vi "EasyDAQx1.vi"() -> ()   [LabVIEW 2011]
panel:
  in  "Show cursor":bool
  out "?":dbl
  out "?":waveform(dbl)(graph)
  in  "Set DAC":bool
  in  "Output (Volts) 2":sgl(slide) caption="Output (Volts)" min=-4.096 max=4.096 step=0.001 scale=-4.096..4.096 scale format="%#.2f"
  out "Numeric":i32
  out "Offsets":dbl[](array[numeric])
  out "Gains":dbl[](array[numeric])
  out "Gain 5":i32
  out "P-Channel":i32
  out "NumBytes":i32
  out "N-channel":i32
  out "NumChannel":i32
  in  "Quit":bool
  out "connected to device":bool
  in  "VISA resource Input":refnum<visa-resource-name>
  in  "Rate (ms)":dbl=500.0 min=10.0 max=65535.0 step=10.0
  out "Final Value":dbl
  in  "Offset":dbl
  in  "Gain":dbl
  out "Voltage":dbl
  in  "OK Button":bool
  in  "?":bool
  in  "Range":string(combo)="1"
  in  "Ch-":string(combo)="0"
  in  "Ch+":string(combo)="7"
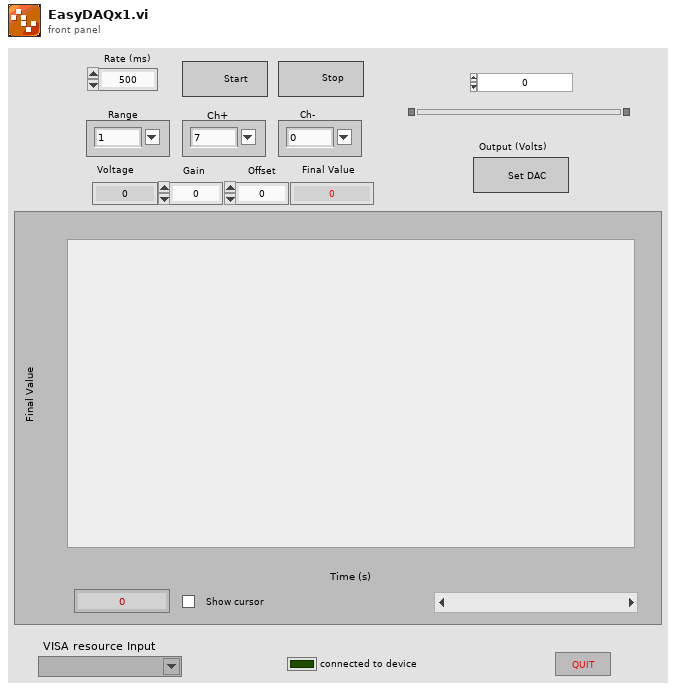
[diagram p1: front panel]
types:
  T1 = enum8{"Enabled", "Disabled", "Disabled and Grayed Out"}
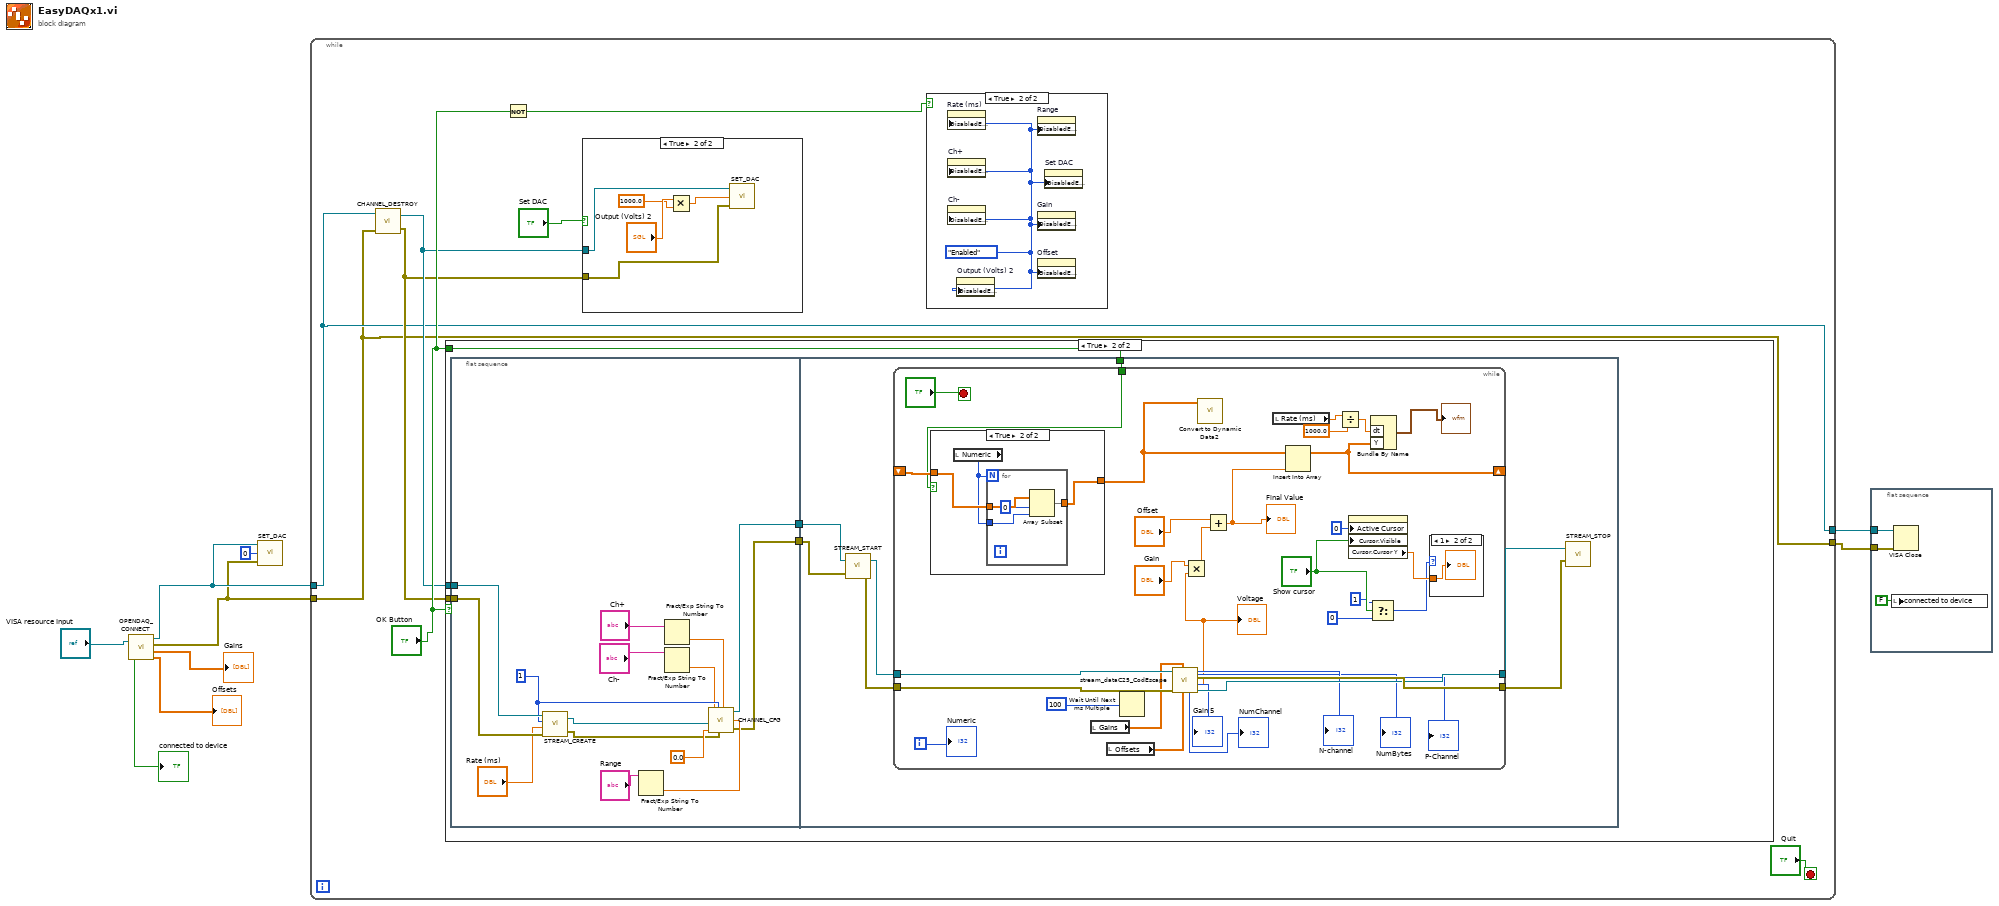
[diagram p0: block diagram]
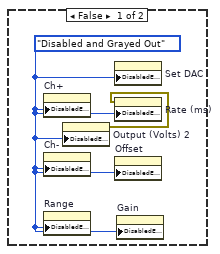
[diagram p3: hidden frame]
diagram:
  n1 = call "OPENDAQ_CONNECT.vi"("VISA resourceINPUT"="VISA resource Input") -> ("connected to device"=→"connected to device":bool, "VISA resource Salida"=w3:refnum<visa-resource-name>, "error out"=w2:errorcluster, "Gains"=→"Gains":dbl[], "Offsets"=→"Offsets":dbl[])
  n2 = call "SET_DAC.vi"("error in (no error)"=w2, "Input"=0, "VISA resource Input"=w3) -> ()  [unwired: 2 out]
  n3 = while {
    tunnel: w3 -> [w11]
    tunnel: w2 -> [w10]
    tunnel: [w11] -> w9
    tunnel: [w10] -> w8
    stop <- "Quit" stop-if-true
    n4 = call "CHANNEL_DESTROY.vi"("error INPUT"=w10, "VISA resource Input"=w11) -> ("error out"=w13:errorcluster, "VISA resource name out"=w14:refnum<visa-resource-name>)  [unwired: 1 in]
    n5 = case shown="True" "OK Button" {
      tunnel: w14 -> [_ w30]
      tunnel: w13 -> [_ w29]
      tunnel: "OK Button" -> [_ w26]
      frame False {
      }
      frame True {
        n6 = flat-sequence {
          tunnel: w30 -> [w45]
          tunnel: w29 -> [w44]
          tunnel: [w32] -> w28
          tunnel: [w31] -> w27
          tunnel: w28 -> [w48]
          tunnel: w27 -> [w47]
          tunnel: w26 -> [w46]
          frame #0 {
            w41 = i8 1 ("Channel")
            n7 = call "STREAM_CREATE.vi"("error in (no error)"=w44, "Period"="Rate (ms)", "Channel"=w41, "VISA resource Input"=w45) -> ("error out"=w39:errorcluster, "VISA resource name out"=w42:refnum<visa-resource-name>)
            n8 = Fract/Exp String To Number(string="Range") -> (number=w33:dbl)  [unwired: 3 in, 1 out]
            n9 = Fract/Exp String To Number(string="Ch+") -> (number=w37:dbl)  [unwired: 3 in, 1 out]
            n10 = Fract/Exp String To Number(string="Ch-") -> (number=w35:dbl)  [unwired: 3 in, 1 out]
            n11 = call "CHANNEL_CFG.vi"("Pchan"=w37, "Channel"=w41, "Nchan"=w35, "VISA resource name"=w42, "error in (no error)"=w39, "Mode"=0.0, "Gain"=w33) -> ("VISA resource name out"=w32:refnum<visa-resource-name>, "error out"=w31:errorcluster)
          }
          frame #1 {
            n12 = call "STREAM_START.vi"("error in (no error)"=w47, "VISA resource name"=w48) -> ("error out"=w52:errorcluster, "VISA resource name out"=w51:refnum<visa-resource-name>)
            n13 = while {
              tunnel: w51 -> [w84]
              tunnel: w52 -> [w83]
              tunnel: [w81] -> w50
              tunnel: [w82] -> w49
              shift-right: [w63] -> _
              shift-left: _ -> [w75]
              tunnel: w46 -> [w71]
              i -> [w69]
              stop <- "?" stop-if-true
              n14 = case shown="True" w71 {
                tunnel: w75 -> [w87 w90]
                tunnel: [w87 w89] -> w70
                frame False {
                }
                frame True {
                  n15 = local read "Numeric"() -> (w88:i32)
                  n16 = for {
                    N: w88 -> [_]
                    tunnel: w90 -> [w94]
                    tunnel: [w92] -> w89
                    tunnel: w88 -> [w91]
                    n17 = Array Subset(array=w94, index=0, length=w91) -> (w92:dbl[])
                  }
                }
              }
              n18 = local read "Gains"() -> (w74:dbl[])
              n19 = local read "Offsets"() -> (w73:dbl[])
              n20 = Wait Until Next ms Multiple(millisecond multiple=u32 100) -> ()  [unwired: 1 out]
              n21 = call "stream_dataC25_CodEscape.vi"("Offsets"=w73, "Gains"=w74, "error out 2"=w83, "VISA resource name out 2"=w84) -> ("VISA resource name out"=w81:refnum<visa-resource-name>, "DATA"=w67:dbl, "P-Channel"=→"P-Channel":i32, "N-channel"=→"N-channel":i32, "NumChannel"=→"NumChannel":i32, "NumBytes"=→"NumBytes":i32, "Gain"=→"Gain 5":i32, "error out"=w82:errorcluster)
              "Voltage" <- w67
              n22 = Multiply(x="Gain", y=w67) -> (x*y=w66:dbl)
              n23 = call "Convert to Dynamic Data2"("Array"=w70) -> ()  [unwired: 3 in, 1 out]
              n24 = Add(x="Offset", y=w66) -> (x+y=w64:dbl)
              "Final Value" <- w64
              n25 = local read "Rate (ms)"() -> (w61:dbl)
              n26 = Insert Into Array(array=w70, new element=w64) -> (w63:dbl[])  [unwired: 1 in]
              n27 = Divide(x=w61, y=1000.0) -> (x/y=w62:dbl)
              n28 = property class="WFGraph (strict)"("Active Cursor"=u32 0, "Cursor.Visible"="Show cursor") -> ("Cursor.Cursor Y"=w56:dbl)  [unwired: 2 in, 2 out]
              n29 = Bundle By Name("dt"=w62, "Y"=w63) -> (→"?":waveform(dbl))  [unwired: 1 in]
              n30 = Select(t=u8 1 ("Disabled"), s="Show cursor", f=u8 0 ("Disabled")) -> (s? t:f=w54:u8)
              n31 = case shown="1" w54 {
                tunnel: w56 -> [_ w86]
                frame 0, Default {
                }
                frame 1 {
                  "?" <- w86
                }
              }
              "Numeric" <- w69
            }
            n32 = call "STREAM_STOP.vi"("error in (no error)"=w49, "VISA resource name"=w50) -> ()  [unwired: 2 out]
          }
        }
      }
    }
    n33 = Not(x="OK Button") -> (.not. x?=w15:bool)
    n34 = case shown="True" "Set DAC" {
      tunnel: w14 -> [_ w22]
      tunnel: w13 -> [_ w21]
      frame False {
      }
      frame True {
        n35 = Multiply(x="Output (Volts) 2", y=sgl 1000.0) -> (x*y=w18:sgl)
        n36 = call "SET_DAC.vi"("error in (no error)"=w21, "Input"=w18, "VISA resource Input"=w22) -> ()  [unwired: 2 out]
      }
    }
    n37 = case shown="True" w15 {
      frame False {
        w23 = T1."Disabled and Grayed Out" ("Disabled")
        n38 = property on="Ch+" class="CmbBox"("DisabledEnum"=w23) -> ()  [unwired: 2 in, 2 out]
        n39 = property on="Ch-" class="CmbBox"("DisabledEnum"=w23) -> ()  [unwired: 2 in, 2 out]
        n40 = property on="Range" class="CmbBox"("DisabledEnum"=w23) -> ()  [unwired: 2 in, 2 out]
        n41 = property on="Output (Volts) 2" class="Slide (strict)"("DisabledEnum"=w23) -> (error out=w24:errorcluster)  [unwired: 2 in, 1 out]
        n42 = property on="Set DAC" class="Bool"("DisabledEnum"=w23) -> ()  [unwired: 2 in, 2 out]
        n43 = property on="Rate (ms)" class="DigNum (strict)"(error in=w24, "DisabledEnum"=w23) -> ()  [unwired: 1 in, 2 out]
        n44 = property on="Offset" class="DigNum (strict)"("DisabledEnum"=w23) -> ()  [unwired: 2 in, 2 out]
        n45 = property on="Gain" class="DigNum (strict)"("DisabledEnum"=w23) -> ()  [unwired: 2 in, 2 out]
      }
      frame True {
        w25 = T1."Enabled" ("Disabled")
        n46 = property on="Rate (ms)" class="DigNum (strict)"("DisabledEnum"=w25) -> ()  [unwired: 2 in, 2 out]
        n47 = property on="Ch+" class="CmbBox"("DisabledEnum"=w25) -> ()  [unwired: 2 in, 2 out]
        n48 = property on="Ch-" class="CmbBox"("DisabledEnum"=w25) -> ()  [unwired: 2 in, 2 out]
        n49 = property on="Output (Volts) 2" class="Slide (strict)"("DisabledEnum"=w25) -> ()  [unwired: 2 in, 2 out]
        n50 = property on="Range" class="CmbBox"("DisabledEnum"=w25) -> ()  [unwired: 2 in, 2 out]
        n51 = property on="Gain" class="DigNum (strict)"("DisabledEnum"=w25) -> ()  [unwired: 2 in, 2 out]
        n52 = property on="Offset" class="DigNum (strict)"("DisabledEnum"=w25) -> ()  [unwired: 2 in, 2 out]
        n53 = property on="Set DAC" class="Bool"("DisabledEnum"=w25) -> ()  [unwired: 2 in, 2 out]
      }
    }
  }
  n54 = flat-sequence {
    tunnel: w9 -> [w97]
    tunnel: w8 -> [w96]
    frame #0 {
      n55 = local write "connected to device"(FALSE ("connected to device")) -> ()
      n56 = VISA Close(VISA resource name=w97, error in (no error)=w96) -> ()  [unwired: 1 out]
    }
  }
